vi "test-trajectory-transform-01.vi"() -> (3 "Test Passed":bool)   [LabVIEW 2019]
uses:
  <vilib>/Rock Robotics/WPI/ThirdParty/JAS_Junk/TrajLib/TRAJECTORY_SPLINE_TYPE_ENUM.ctl
  <vilib>/Rock Robotics/WPI/ThirdParty/JAS_Junk/TrajLib/Rotation_CreateAngle.vi
  <vilib>/Rock Robotics/WPI/ThirdParty/JAS_Junk/TrajLib/Translation_Equals.vi
  <vilib>/Rock Robotics/WPI/ThirdParty/JAS_Junk/TrajLib/Rotation_Equals.vi
  <vilib>/Rock Robotics/WPI/ThirdParty/JAS_Junk/TrajLib/Util_CalcDist.vi
  <vilib>/Rock Robotics/WPI/ThirdParty/JAS_Junk/TrajLib/Trajectory_Library.lvlib
panel:
  out "XY Graph":cluster{dbl[], dbl[]}[](graph)
  out "ShapeOkay":bool
  out "Starting Pose Okay":bool
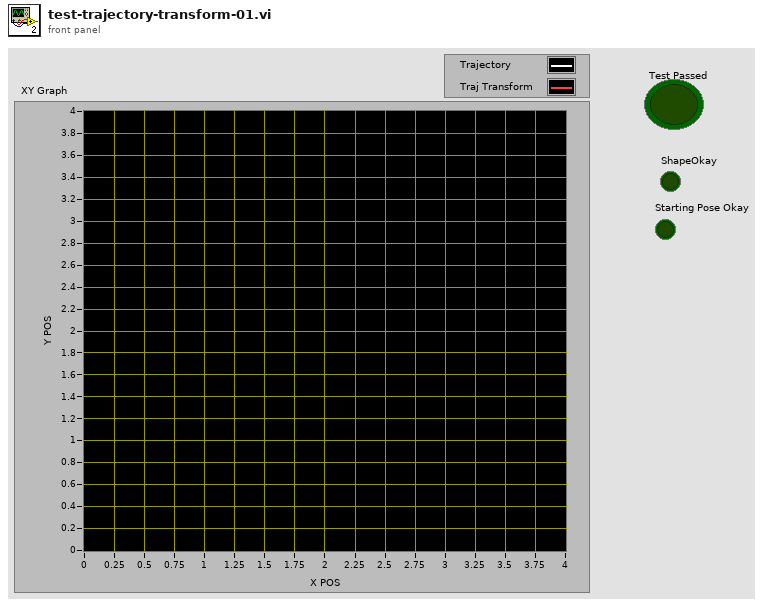
[diagram p1: front panel]
types:
  T1 = typedef "Trajectory_Library.lvlib/TRAJECTORY_SPLINE_TYPE_ENUM.ctl" = enum16{"Cubic", "Cubic With Weights", "Quintic", "Quintic With Weights"}
  T2 = typedef "Trajectory_Library.lvlib/WEIGHTED_WAYPOINT.ctl" = cluster{"TRANSLATION":T3, "ROTATION":T4, "SCALAR":dbl}
  T3 = typedef "Trajectory_Library.lvlib/TRANSLATION2D.ctl" = cluster{"X":dbl, "Y":dbl}
  T4 = typedef "Trajectory_Library.lvlib/ROTATION2D.ctl" = cluster{"VALUE":dbl, "COS":dbl, "SIN":dbl}
  T5 = typedef "Trajectory_Library.lvlib/TRAJ_CONFIG.ctl" = cluster{"MaxVelocity":dbl, "Max Acceleration":dbl, "StartVelocity":dbl, "End Velocity":dbl, "Reversed":bool, "DiffDrKineConstntDefined":bool, "CentAcellConstntDefined":bool, "DiffDrVoltConstntDefined":bool, "DIFF_DRIVE_KINE_CONSTRAINT":T6, "CENTRIPETAL_ACCEL_CONSTRAINT":T8, "SwerveDrKineConstntDefined":bool, "SWERVE_DRIVE_KINE_CONSTRAINT":T9, "DIFF_DRIVE_VOLTAGE_CONSTRAINT":T12, "MECANUM_DRIVE_KINE_CONSTRAINT":T14, "MecanumDrKineConstntDefined":bool}
  T6 = typedef "Trajectory_Library.lvlib/TRAJ_CONSTRAINT_DIIF_DRIVE_KINEMATICS.ctl" = cluster{"Max Speed (M/S)":dbl, "DIFF_DRIVE_KINEMATICS":T7, "Max Accel (M/S2)":dbl}
  T7 = typedef "Trajectory_Library.lvlib/DIFF_DRIVE_KINEMATICS.ctl" = cluster{"TrackWidth_Meters":dbl}
  T8 = typedef "Trajectory_Library.lvlib/TRAJ_CONSTRAINT_CENTRIPETAL_ACCEL.ctl" = cluster{"Max Cent Accel":dbl}
  T9 = typedef "Trajectory_Library.lvlib/TRAJ_CONSTRAINT_SWERVE_DRIVE_KINEMATICS.ctl" = cluster{"Max Speed (M/S)":dbl, "SwerveKinematics":T10}
  T10 = typedef "Trajectory_Library.lvlib/SWERVE_DRIVE_KINEMATICS.ctl" = cluster{"NumModules":i32, "InverseKinematics":T11, "ForwardKinematics":T11, "Modules":T3[], "PrevCoR":T3}
  T11 = typedef "NI_Matrix.lvlib/RealMatrix.ctl" = dbl[][]
  T12 = typedef "Trajectory_Library.lvlib/TRAJ_CONSTRAINT_DIIF_DRIVE_VOLTAGE.ctl" = cluster{"Max Voltage":dbl, "DIFF_DRIVE_KINEMATICS":T7, "SIMPLE_MOTOR_FF":T13}
  T13 = typedef "Trajectory_Library.lvlib/SIMPLE_MOTOR_FF.ctl" = cluster{"Ks":dbl, "Kv":dbl, "Ka":dbl}
  T14 = typedef "Trajectory_Library.lvlib/TRAJ_CONSTRAINT_MECA_DRIVE_KINEMATICS.ctl" = cluster{"Max Speed (M/S)":dbl, "MECA_DRIVE_KINEMATICS":T15}
  T15 = typedef "Trajectory_Library.lvlib/MECA_DRIVE_KINEMATICS.ctl" = cluster{"FrontLeft":T3, "FrontRight":T3, "RearLeft":T3, "RearRight":T3, "InverseKinematics":T11, "ForwardKinematics":T11, "PrevCoR":T3}
  T16 = typedef "Trajectory_Library.lvlib/TRAJECTORY.ctl" = cluster{"TotalTImeSecs":dbl, "States":T17[]}
  T17 = typedef "Trajectory_Library.lvlib/TRAJ_STATE.ctl" = cluster{"TimeSeconds":dbl, "Velocity":dbl, "Acceleration":dbl, "POSE":T18, "Curvature":dbl}
  T18 = typedef "Trajectory_Library.lvlib/POSE2D.ctl" = cluster{"TRANSLATION":T3, "ROTATION":T4}
  T19 = typedef "Trajectory_Library.lvlib/TRANSFORM2D.ctl" = cluster{"TRANSLATION":T3, "ROTATION":T4}
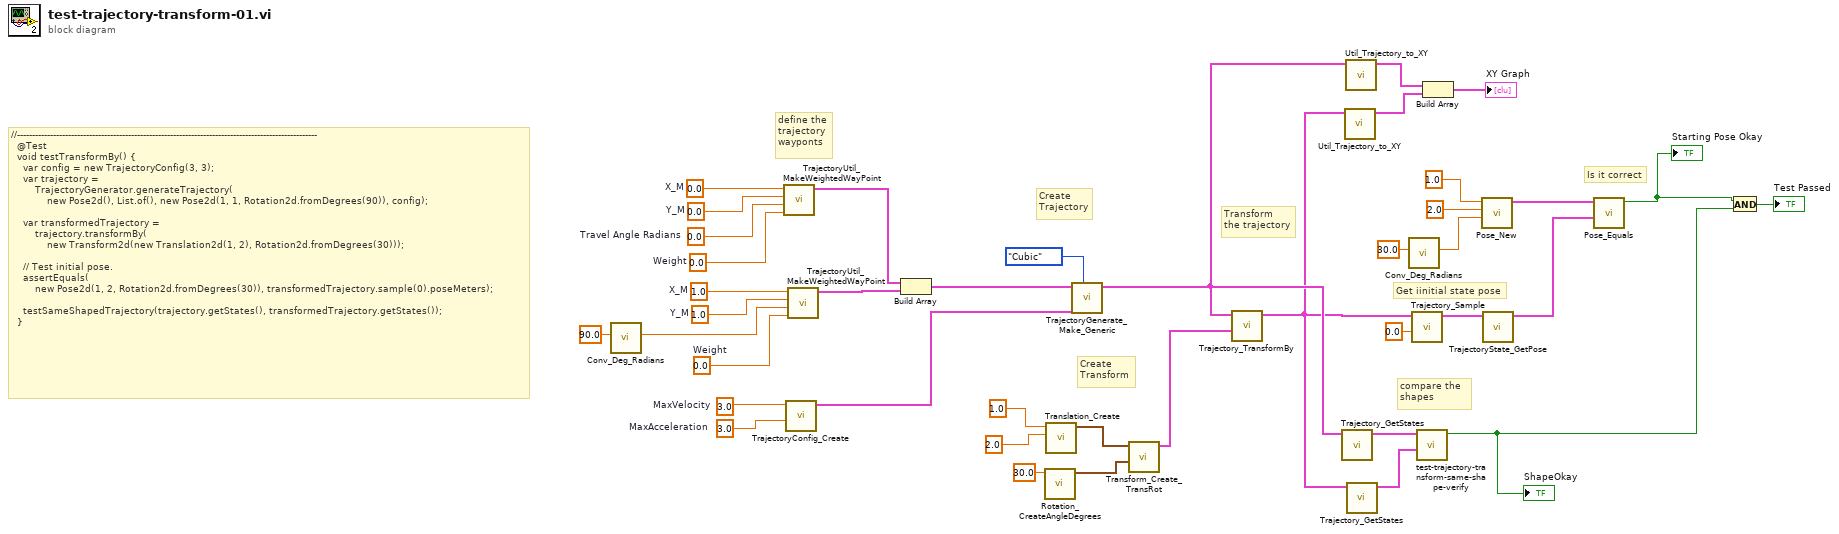
[diagram p0: block diagram]
diagram:
  w39 = 1.0  # X_M
  w38 = 1.0  # Y_M
  w37 = 0.0  # Weight
  w36 = 0.0  # X_M
  w35 = 0.0  # Y_M
  w34 = 0.0  # Travel Angle Radians
  w33 = 0.0  # Weight
  w32 = 3.0  # MaxVelocity
  w31 = 3.0  # MaxAcceleration
  # "define the\ntrajectory\nwayponts"
  # "Is it correct"
  # "Get iinitial state pose"
  # "compare the \nshapes"
  # "Transform\nthe trajectory"
  # "Create\nTransform"
  # "Create\nTrajectory"
  # "//----------------------------------------------------------------------------------------------------\n  @Test\n  void testTransformBy() {\n    var config = new TrajectoryConfig(3, 3);\n    var trajectory =\n        TrajectoryGenerator.generateTrajectory(\n            new Pose2d(), List.of(), new Pose2d(1, 1, Rotation2d.fromDegrees(90)), config);\n\n    var transformedTrajectory =\n        trajectory.transformBy(\n            new Transform2d(new Translation2d(1, 2), Rotation2d.fromDegrees(30)));\n\n    // Test initial pose.\n    assertEquals(\n        new Pose2d(1, 2, Rotation2d.fromDegrees(30)), transformedTrajectory.sample(0).poseMeters);\n\n    testSameShapedTrajectory(trajectory.getStates(), transformedTrajectory.getStates());\n  }"
  n1 = call <vilib>:"Conv_Deg_Radians.vi"("Degress"=90.0) -> ("Radians"=w25:dbl)  [unwired: 10 in]
  n2 = call <vilib>:"TrajectoryUtil_MakeWeightedWayPoint.vi"("Weight"=w33, "Travel Angle Radians"=w34, "Y_M"=w35, "X_M"=w36) -> ("WEIGHTED_WAYPOINT"=w27:T2)  [unwired: 7 in]
  n3 = call <vilib>:"TrajectoryConfig_Create.vi"("MaxAcceleration"=w31, "MaxVelocity"=w32) -> ("TRAJECTORY_CONFIG"=w30:T5)  [unwired: 9 in]
  n4 = call <vilib>:"TrajectoryUtil_MakeWeightedWayPoint.vi"("Weight"=w37, "Travel Angle Radians"=w25, "Y_M"=w38, "X_M"=w39) -> ("WEIGHTED_WAYPOINT"=w40:T2)  [unwired: 7 in]
  n5 = Build Array(w27, w40) -> (w28:T2[])
  n6 = call <vilib>:"Rotation_CreateAngleDegrees.vi"("Angle_Degrees"=30.0) -> ("ROTATION"=w23:T4)  [unwired: 10 in]
  n7 = call <vilib>:"Translation_Create.vi"("Y"=2.0, "X"=1.0) -> ("TRANSLATION"=w24:T3)  [unwired: 9 in]
  n8 = call <vilib>:"TrajectoryGenerate_Make_Generic.vi"("Spline Type"=TRAJECTORY_SPLINE_TYPE_ENUM."Cubic", "traj_config"=w30, "WeightedWayPoints"=w28) -> ("TRAJECTORY"=w2:T16)  [unwired: 7 in, 1 out]
  n9 = call <vilib>:"Transform_Create_TransRot.vi"("ROTATION"=w23, "TRANSLATION"=w24) -> ("TRANSFORM"=w19:T19)  [unwired: 9 in]
  n10 = call <vilib>:"Trajectory_TransformBy.vi"("TRANSFORM"=w19, "InputTRAJECTORY"=w2) -> ("outputTRAJECTORY"=w1:T16)  [unwired: 9 in]
  n11 = call <vilib>:"Trajectory_GetStates.vi"("TRAJECTORY"=w2) -> ("States"=w18:T17[])  [unwired: 10 in]
  n12 = call <vilib>:"Util_Trajectory_to_XY.vi"("TRAJECTORY"=w1) -> ("outArrayXY"=w4:cluster{dbl[], dbl[]})  [unwired: 10 in]
  n13 = call <vilib>:"Util_Trajectory_to_XY.vi"("TRAJECTORY"=w2) -> ("outArrayXY"=w5:cluster{dbl[], dbl[]})  [unwired: 10 in]
  n14 = call <vilib>:"Trajectory_GetStates.vi"("TRAJECTORY"=w1) -> ("States"=w17:T17[])  [unwired: 10 in]
  n15 = call <vilib>:"Conv_Deg_Radians.vi"("Degress"=30.0) -> ("Radians"=w11:dbl)  [unwired: 10 in]
  n16 = call <vilib>:"Trajectory_Sample.vi"("Time"=0.0, "InputTRAJECTORY"=w1) -> ("OutputTRAJ_STATE"=w15:T17)  [unwired: 9 in]
  n17 = call "test-trajectory-transform-same-shape-verify.vi"("TrajStates2"=w17, "TrajStates1"=w18) -> ("SameShape"=w7:bool)  [unwired: 9 in]
  "ShapeOkay" <- w7
  n18 = Build Array(w5, w4) -> (→"XY Graph":cluster{dbl[], dbl[]}[])
  n19 = call <vilib>:"Pose_New.vi"("Heading"=w11, "Y"=2.0, "X"=1.0) -> ("out POSe"=w10:T18)  [unwired: 8 in]
  n20 = call <vilib>:"TrajectoryState_GetPose.vi"("TRAJ_STATE"=w15) -> ("TrajStatePose"=w9:T18)  [unwired: 10 in]
  n21 = call <vilib>:"Pose_Equals.vi"("other POSE"=w9, "in POSE"=w10) -> ("Equals"=w8:bool)  [unwired: 9 in]
  "Starting Pose Okay" <- w8
  n22 = And(x=w8, y=w7) -> (x .and. y?=→"Test Passed":bool)
